vi "Agilent 87XX Series Exceed Max Meas.vi"() -> ()   [LabVIEW 2018]
doc: "This example for the HP8753B Network Analyzer demonstrates how to use the driver to take a series of measurements over a range of values, thus allowing the operator to take more than the maximum of 1601 measurements. \n The measurement range is broken up into a number of segments set by the user. Each segment is configured, triggered and read seperately. The data is then put together into one big array and graphed.\n This VI assumes that all the configuring except setting the start and stop frequencies and measurement format have been done before the VI is run."
uses:
  Agilent 87XX Series.lvlib
panel:
  out "graphical display 1":cluster{dbl, dbl}[](graph)
  in  "display format":u16(ring) items=["log magnitude", "phase", "delay", "Smith chart", "polar", "linear magnitude", "standing wave ratio", "real", "imaginary"]
  out "data values":cluster{"real / stim":dbl, "imag / resp":dbl}[](array[cluster]) {"imag / resp" format="%.4e"; "real / stim" format="%.4e"}
  in  "error in (no error)":errorcluster
  out "error out":errorcluster
  out "VISA resource name out":refnum<visa-resource-name>
  in  "VISA resource name":refnum<visa-resource-name>
  in  "num points / segment":u16(ring)=5 items=["3", "11", "21 ('20) / 26 ('53)", "51", "101", "201", "401", "801", "1601"]
  in  "num of segments":i32=18
  in  "stop (GHz)":dbl=10.0 format="%.2e"
  in  "start (GHz)":dbl=1.0 format="%.2e"
  # "© 2005 National Instruments.  ALL RIGHTS RESERVED."
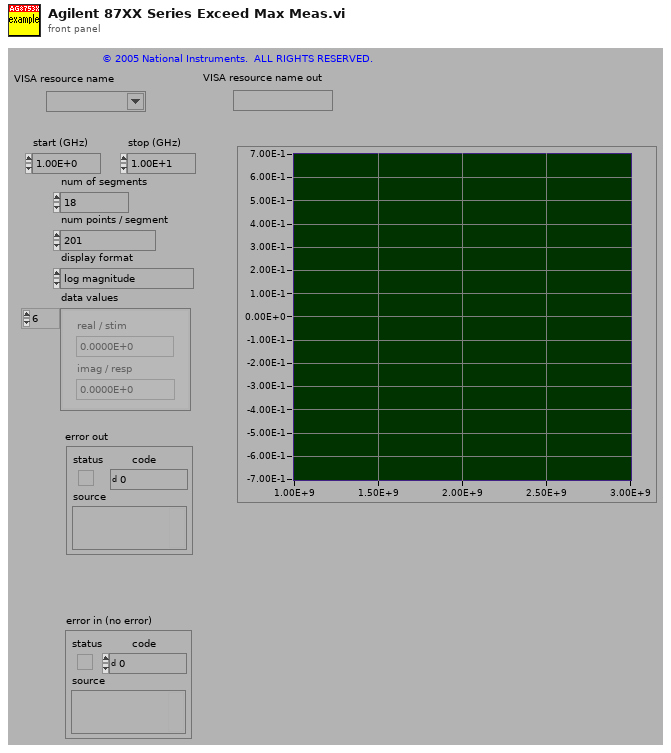
[diagram p1: front panel]
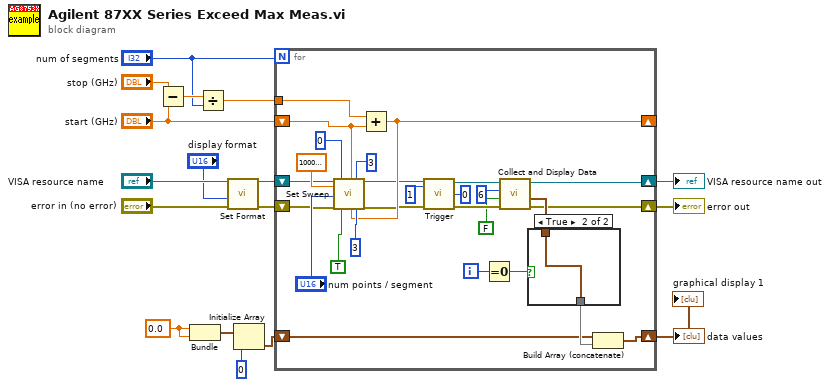
[diagram p0: block diagram]
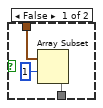
[diagram p2: hidden frame]
diagram:
  w12 = 0.0
  n1 = Subtract(x="stop (GHz)", y="start (GHz)") -> (x-y=w17:dbl)
  n2 = Bundle(w12, w12) -> (w11:cluster{dbl, dbl})  [unwired: 1 in]
  n3 = Divide(x=w17, y="num of segments") -> (x/y=w15:dbl)
  n4 = call "Set Format.vi"("error in (no error)"="error in (no error)", "format (0 : log mag)"="display format", "VISA resource name"="VISA resource name") -> ("error out"=w3:errorcluster, "VISA resource name out"=w6:refnum<visa-resource-name>)  [unwired: 7 in]
  n5 = Initialize Array(w11, 0) -> (w9:cluster{dbl, dbl}[])
  n6 = for {
    N: "num of segments" -> [_]
    shift-right: [w37] -> _
    shift-left: "start (GHz)" -> [w18]
    tunnel: w15 -> [w38]
    shift-right: [w19] -> w1
    shift-left: w9 -> [w24]
    shift-right: [w21] -> w8
    shift-left: w6 -> [w23]
    shift-right: [w20] -> w7
    shift-left: w3 -> [w22]
    i -> [w28]
    n7 = Add(x=w38, y=w18) -> (x+y=w37:dbl)
    n8 = call "Set Sweep.vi"("VISA resource name"=w23, "CW freq (Hz)"=1000000000.0, "num points"="num points / segment", "error in (no error)"=w22, "sweep type (0 : linear)"=u16 0, "t: start/stop  f: center/span"=TRUE, "start/center"=w18, "stop/span"=w37, "start/center units (1 : Hz/dBm)"=u16 3, "stop/span units (0 : Hz/dBm)"=u16 3) -> ("VISA resource name out"=w36:refnum<visa-resource-name>, "error out"=w35:errorcluster)  [unwired: 8 in]
    n9 = call "Trigger.vi"("trigger (1 : single)"=u16 1, "error in (no error)"=w35, "trigger source (0 : ext trig off)"=u16 0, "VISA resource name"=w36) -> ("error out"=w31:errorcluster, "VISA resource name out"=w32:refnum<visa-resource-name>)  [unwired: 6 in]
    n10 = Equal To 0?(x=w28) -> (x = 0?=w27:bool)
    n11 = call "Collect and Display Data.vi"("error in (no error)"=w31, "save to file"=FALSE, "data type (6 : formatted data)"=u16 6, "VISA resource name"=w32) -> ("error out"=w20:errorcluster, "data values"=w26:cluster{"real / stim":dbl, "imag / resp":sgl}[], "VISA resource name out"=w21:refnum<visa-resource-name>)  [unwired: 4 in, 1 out]
    n12 = case shown="True" w27 {
      tunnel: w26 -> [w47 w48]
      tunnel: [w45 w48] -> w25
      frame False {
        n13 = Array Subset(array=w47, index=1) -> (w45:cluster{"real / stim":dbl, "imag / resp":sgl}[])  [unwired: 1 in]
      }
      frame True {
      }
    }
    n14 = Build Array (concatenate)(w24, w25) -> (w19:cluster{"real / stim":dbl, "imag / resp":dbl}[])
  }
  "VISA resource name out" <- w8
  "error out" <- w7
  "data values" <- w1
  "graphical display 1" <- w1
